vi "Core Write U8 FIFO.vi"(8 "error in (no error)":errorcluster, 10 "Data In":T1[](array[typedef]), 11 "CIFFIFO in":refnum<class "CIF_CIPC_Fifo_DAQ.lvclass">) -> (0 "error out":errorcluster, 2 "Data Out":T1[](array[typedef]), 3 "CIFFIFO out":refnum<class "CIF_CIPC_Fifo_DAQ.lvclass">)   [LabVIEW 2021, in "CIF_CIPC_Fifo_DAQ.lvclass"]
uses:
  CIF_CIPC_Fifo_DAQ.lvclass
  D:/dev/Packages/CIF_Channels_Core/src/CIFChannels/CIFChannels.lvclass
  D:/dev/Packages/CIF_Channels_Core/src/CIPC_Channels/CIF_CIPC_Chan/CIF_CIPC_Chn.lvclass
  CIFChannels/CIFChannels.lvclass/CIFChannels.ctl
  CIF_CIPC_Chan/CIF_CIPC_Chn.lvclass/CIF_CIPC_Chn.ctl
  <vilib>/CIF Foundation/CIF CIPC/TypeDefs/Partial Write Configuration.ctl
  <vilib>/CIF Foundation/CIF Utilities/Statistics/I64/Stats_I64_CIF_U.lvclass/Stats_I64_CIF_U.ctl
  1bad10da-a98b-49ee-b03a-18b497e396df.vi
  70f860b1-5d4a-43dc-b0c2-c9446e8447f7.vi
  40f8d1bb-2a62-444a-8ee6-d4d6c496dc12.vi
  CIFChannels/Accessors/Read FIFO Header.vi
  <vilib>/CIF Foundation/CIF Utilities/Statistics/I64/X1 minus X0.vi
  <vilib>/CIF Foundation/CIF Utilities/Time/System Time/Get System Time.vi
  <vilib>/CIF Foundation/CIF CIPC/SubVIs/Check Error.vi
  <vilib>/CIF Foundation/CIF CIPC/SubVIs/Notify Of New Write.vi
  <vilib>/CIF Foundation/CIF CIPC/SubVIs/Get dll Path.vi
  <vilib>/CIF Foundation/CIF CIPC/SubVIs/Get Element Write Position.vi
  <vilib>/CIF Foundation/CIF Utilities/Statistics/I64/X1 minus X0.vi/dfabcf33-0dbc-4041-80a5-3dc0c86d2989.vi
  <vilib>/CIF Foundation/CIF Utilities/Time/System Time/LabVIEW Time to TAI Time.vi
  <vilib>/CIF Foundation/CIF Utilities/Statistics/I64/X1 minus X0.vi/dfabcf33-0dbc-4041-80a5-3dc0c86d2989.vi/9eb60a9a-770f-4d2d-8b3f-8465c267ecc9.vi
  <vilib>/Utility/error.llb/Trim Whitespace.vi
  <vilib>/Utility/error.llb/Error Cluster From Error Code.vi
  CIF_CIPC_Fifo_DAQ.lvclass/CIF_CIPC_Fifo_DAQ.ctl
  CIFChannels/CIFChannels.lvclass
  CIF_CIPC_Chan/CIF_CIPC_Chn.lvclass
  <vilib>/CIF Foundation/CIF CIPC/CIF_NI_CIPC.lvlib
  2677c56d-ef03-42ec-8b9a-5383cd517bf2.vi
  b87aee52-4999-4b0a-a6e0-2114ae1ac292.vi
  1797c2fb-4c7a-4e01-b5c1-3e65a4947bb5.vi
  D:/dev/Packages/CIF_Channels_Core/src/CIPC_Channels/FIFO_DAQ/CIF_CIPC_Fifo_DAQ.lvclass
  ChannelCommon/typedef/Datatype Waveform.ctl
  ChannelCommon/ChannelCommon.lvlib
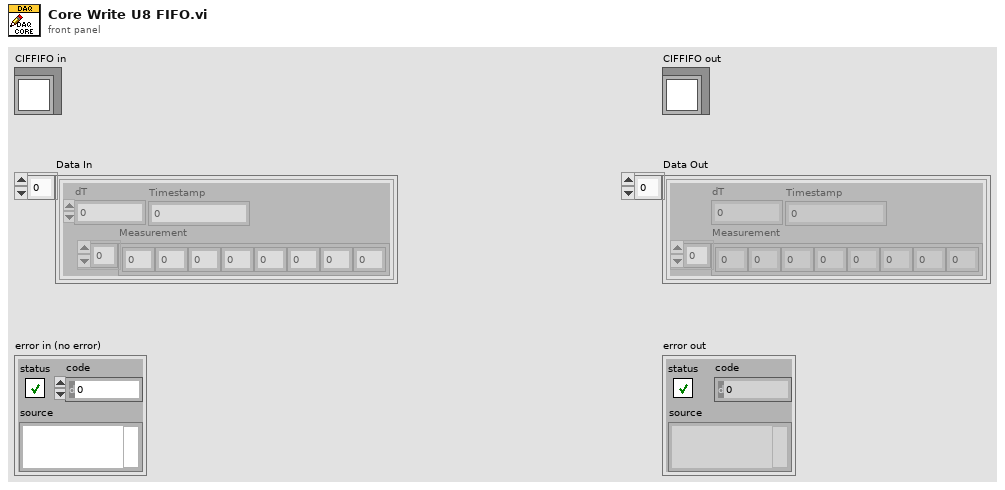
[diagram p1: front panel]
types:
  T1 = typedef "ChannelCommon.lvlib/Datatype Waveform.ctl" = cluster{"Measurement":dbl[], "dT":dbl, "Timestamp":i64}
  T2 = typedef "CIF_NI_CIPC.lvlib/Partial Write Configuration.ctl" = cluster{"Start Offset (bytes)":u32, "Total Length (bytes)":u32, "Last Write":bool, "Get Write Position":bool, "Notify Readers":bool}
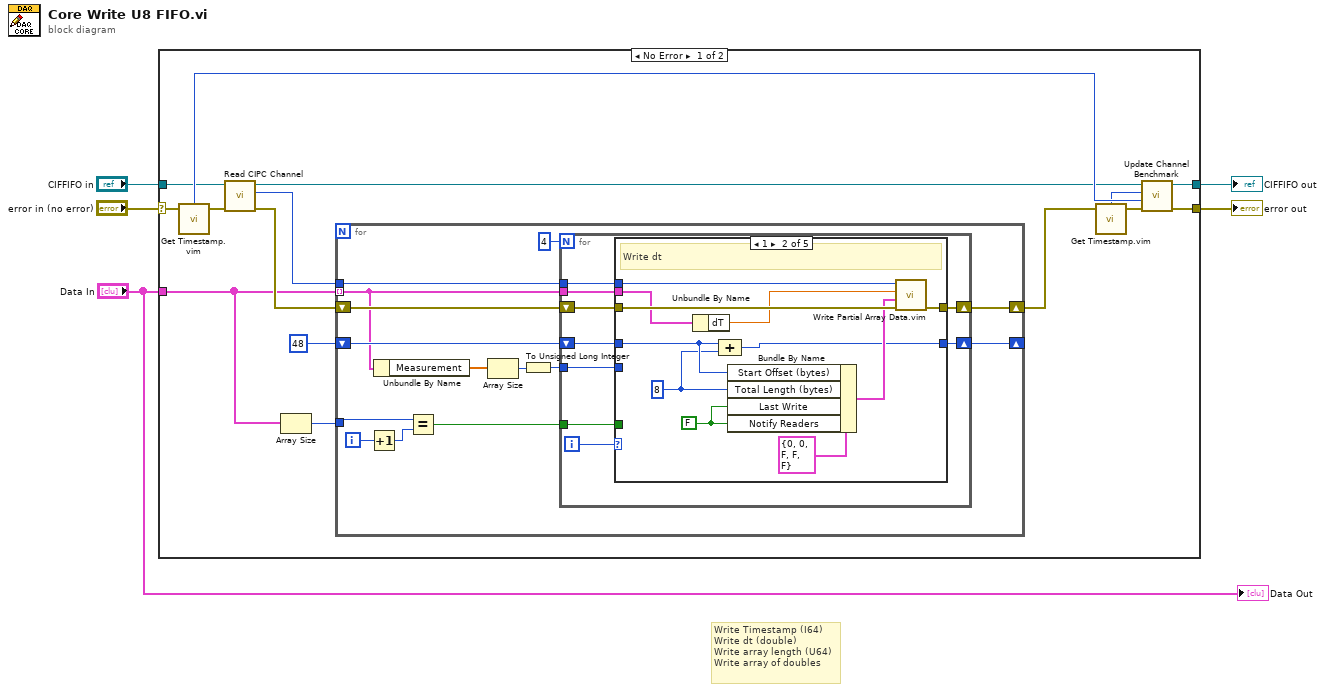
[diagram p0: block diagram]
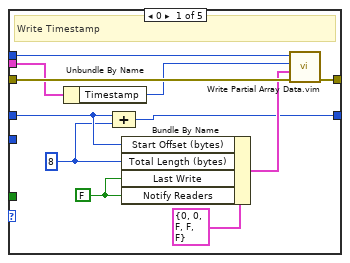
[diagram p2: hidden frame]
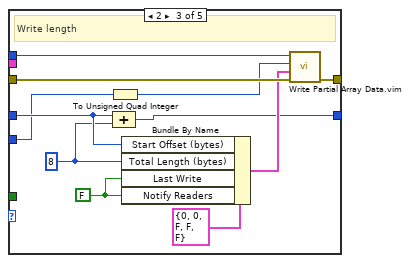
[diagram p3: hidden frame]
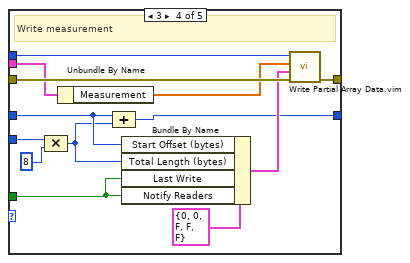
[diagram p4: hidden frame]
diagram:
  # "Write Timestamp (I64)\nWrite dt (double)\nWrite array length (U64)\nWrite array of doubles"
  n1 = case shown="No Error" "error in (no error)" {
    selector: "error in (no error)" -> [w16 w93]
    tunnel: [w20 w93] -> w4
    tunnel: [w19 w92] -> w2
    tunnel: "CIFFIFO in" -> [w10 w92]
    tunnel: "Data In" -> [w7 _]
    frame No Error {
      n2 = call "Get Timestamp.vim"("Anything in"=w16) -> ("Time (ns)"=w18:i64, "Anything out"=w9:errorcluster)  [unwired: 2 in]
      n3 = call "Read CIPC Channel.vi"("error in (no error)"=w9, "CIFTag in"=w10) -> ("error out"=w12:errorcluster, "CIPC Channel"=w13:u64, "CIFTag out"=w14:refnum<class "CIF_CIPC_Fifo_DAQ.lvclass">)  [unwired: 7 in]
      n4 = Array Size(array=w7) -> (size(s)=w6:i32)
      n5 = for {
        tunnel: w13 -> [w34]
        tunnel: w7 -> [w23] mode=indexing
        shift-right: [w33] -> w11
        shift-left: w12 -> [w24]
        shift-right: [w28] -> _
        shift-left: u32 48 ("y") -> [w32]
        tunnel: w6 -> [w30]
        i -> [w31]
        n6 = Increment(x=w31) -> (x+1=w29:i32)
        n7 = Unbundle By Name(w23) -> ("Measurement"=w25:dbl[])
        n8 = Equal?(x=w30, y=w29) -> (x = y?=w27:bool)
        n9 = Array Size(array=w25) -> (size(s)=w26:i32)
        n10 = To Unsigned Long Integer(number=w26) -> (unsigned 32bit integer=w22:u32)
        n11 = for {
          N: 4 -> [_]
          tunnel: w34 -> [w43]
          tunnel: w23 -> [w40]
          shift-right: [w41] -> w33
          shift-left: w24 -> [w42]
          shift-right: [w37] -> w28
          shift-left: w32 -> [w39]
          tunnel: w27 -> [w36]
          tunnel: w22 -> [w35]
          i -> [w38]
          n12 = case shown="1" w38 {
            tunnel: w43 -> [w54 w65 w76 w89 _]
            tunnel: w42 -> [w53 w64 w75 w88 w91]
            tunnel: [w52 w63 w74 w87 w91] -> w41
            tunnel: w40 -> [w46 w57 _ w82 _]
            tunnel: w39 -> [w49 w60 w71 w84 w90]
            tunnel: [w48 w59 w70 w83 w90] -> w37
            tunnel: w36 -> [_ _ _ w80 _]
            tunnel: w35 -> [_ _ w67 w79 _]
            frame 0 {
              w45 = FALSE ("Last Write")
              w47 = u32 8 ("Total Length (bytes)")
              # "Write Timestamp"
              n13 = Unbundle By Name(w46) -> ("Timestamp"=w44:i64)
              n14 = Compound Arithmetic op=ADD(w49, w47) -> (w48:u32)
              n15 = Bundle By Name(cluster=T2 {"Start Offset (bytes)"=0, "Total Length (bytes)"=0, "Last Write"=FALSE, "Get Write Position"=FALSE, "Notify Readers"=FALSE} ("Partial Write Configuration"), "Start Offset (bytes)"=w49, "Total Length (bytes)"=w47, "Last Write"=w45, "Notify Readers"=w45) -> (w50:T2)
              n16 = call "Write Partial Array Data.vim"("error in (no error)"=w53, "Partial Write Configuration"=w50, "Data in"=w44, "CIPC Reference in"=w54) -> ("error out"=w52:errorcluster)  [unwired: 4 in, 3 out]
            }
            frame 1 {
              w56 = FALSE ("Last Write")
              w58 = u32 8 ("Total Length (bytes)")
              # "Write dt"
              n17 = Unbundle By Name(w57) -> ("dT"=w55:dbl)
              n18 = Compound Arithmetic op=ADD(w60, w58) -> (w59:u32)
              n19 = Bundle By Name(cluster=T2 {"Start Offset (bytes)"=0, "Total Length (bytes)"=0, "Last Write"=FALSE, "Get Write Position"=FALSE, "Notify Readers"=FALSE} ("Partial Write Configuration"), "Start Offset (bytes)"=w60, "Total Length (bytes)"=w58, "Last Write"=w56, "Notify Readers"=w56) -> (w61:T2)
              n20 = call "Write Partial Array Data.vim"("error in (no error)"=w64, "Partial Write Configuration"=w61, "Data in"=w55, "CIPC Reference in"=w65) -> ("error out"=w63:errorcluster)  [unwired: 4 in, 3 out]
            }
            frame 2 {
              w68 = FALSE ("Last Write")
              w69 = u32 8 ("Total Length (bytes)")
              # "Write length"
              n21 = To Unsigned Quad Integer(1:w67) -> (0:w66:u64)
              n22 = Compound Arithmetic op=ADD(w71, w69) -> (w70:u32)
              n23 = Bundle By Name(cluster=T2 {"Start Offset (bytes)"=0, "Total Length (bytes)"=0, "Last Write"=FALSE, "Get Write Position"=FALSE, "Notify Readers"=FALSE} ("Partial Write Configuration"), "Start Offset (bytes)"=w71, "Total Length (bytes)"=w69, "Last Write"=w68, "Notify Readers"=w68) -> (w72:T2)
              n24 = call "Write Partial Array Data.vim"("error in (no error)"=w75, "Partial Write Configuration"=w72, "Data in"=w66, "CIPC Reference in"=w76) -> ("error out"=w74:errorcluster)  [unwired: 4 in, 3 out]
            }
            frame 3 {
              # "Write measurement"
              n25 = Compound Arithmetic op=MULTIPLY(w79, u32 8 ("Total Length (bytes)")) -> (w77:u32)
              n26 = Unbundle By Name(w82) -> ("Measurement"=w81:dbl[])
              n27 = Compound Arithmetic op=ADD(w84, w77) -> (w83:u32)
              n28 = Bundle By Name(cluster=T2 {"Start Offset (bytes)"=0, "Total Length (bytes)"=0, "Last Write"=FALSE, "Get Write Position"=FALSE, "Notify Readers"=FALSE} ("Partial Write Configuration"), "Start Offset (bytes)"=w84, "Total Length (bytes)"=w77, "Last Write"=w80, "Notify Readers"=w80) -> (w85:T2)
              n29 = call "Write Partial Array Data.vim"("error in (no error)"=w88, "Partial Write Configuration"=w85, "Data in"=w81, "CIPC Reference in"=w89) -> ("error out"=w87:errorcluster)  [unwired: 4 in, 3 out]
            }
            frame 4, Default {
              # "Default"
            }
          }
        }
      }
      n30 = call "Get Timestamp.vim"("Anything in"=w11) -> ("Time (ns)"=w17:i64, "Anything out"=w15:errorcluster)  [unwired: 2 in]
      n31 = call "Update Channel Benchmark.vi"("error in (no error)"=w15, "X0"=w18, "X1"=w17, "CIFChannels in"=w14) -> ("error out"=w20:errorcluster, "CIFChannels out"=w19:refnum<class "CIF_CIPC_Fifo_DAQ.lvclass">)  [unwired: 6 in]
    }
    frame Error {
    }
  }
  "error out" <- w4
  "CIFFIFO out" <- w2
  "Data Out" <- "Data In"
